vi "Logic_Add_SPI_Analyzer.vi"(4 "error in (no error)":errorcluster, 5 "Analyzer Settings":T1={"MOSI Channel"=0, "MISO Channel"=1, "CLOCK Channel"=2, "ENABLE Channel"=3, "Bits per Transfer"="8 Bits per Transfer (Standard)"}, 6 "Analyzer Label":string="Test Analyzer", 7 "Session Ref In":T2) -> (0 "error out":errorcluster, 3 "Session Ref Out":T2)   [LabVIEW 2023]
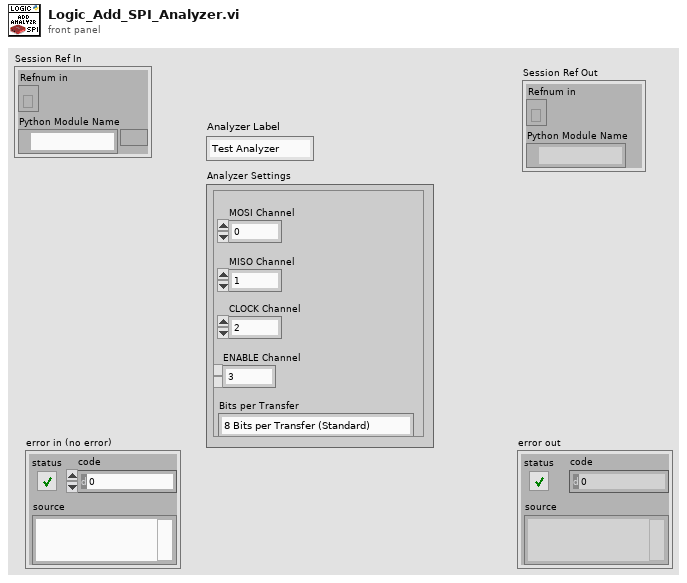
[diagram p1: front panel]
types:
  T1 = cluster{"MOSI Channel":i32, "MISO Channel":i32, "CLOCK Channel":i32, "ENABLE Channel":i32, "Bits per Transfer":string}
  T2 = cluster{"Refnum in":refnum<k35>, "Python Module Name":path}
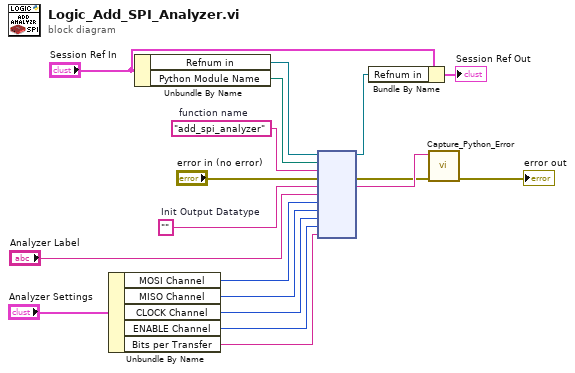
[diagram p0: block diagram]
diagram:
  w17 = "add_spi_analyzer"  # function name
  w16 = ""  # Init Output Datatype
  n1 = Unbundle By Name("Analyzer Settings") -> ("MOSI Channel"=w9:i32, "MISO Channel"=w8:i32, "CLOCK Channel"=w7:i32, "ENABLE Channel"=w6:i32, "Bits per Transfer"=w5:string)
  n2 = Unbundle By Name("Session Ref In") -> ("Refnum in"=w15:refnum<k35>, "Python Module Name"=w14:path)
  n3 = node(w15, w14, w17, "error in (no error)", w16, "Analyzer Label", w9, w8, w7, w6, w5) -> (w12:refnum<k35>, w2:errorcluster, w3:string)  [unwired: 6 in, 2 out]
  n4 = Bundle By Name(cluster="Session Ref In", "Refnum in"=w12) -> (→"Session Ref Out":T2)
  n5 = call "Capture_Python_Error.vi"("error in (no error)"=w2, "Error Message (start with ERROR)"=w3) -> ("error out"=→"error out":errorcluster)  [unwired: 9 in]
